vi "Telemetry Downlink Templates.vi"(11 "Command":T1 items=["Get xPG Status", "xPG Stimulation", "Select Program", "Increment Program Amplitude", "Decrement Program Amplitude", "Get PoP Constants", "Get PPC Constants", "Get Program Names", "Set Pulse Amplitude", "Increment Pulse Amplitude", "Decrement Pulse Amplitude", "Get Pulse Widths", "Set Pulse Widths", "Increment Pulse Width", "Decrement Pulse Width", "Get Program Frequency", "Set Program Frequency", "Increment Program Frequency", "Decrement Program Frequency", "Inject Event", "Charging Control", "Get xPG Identity", "Set xPG Identity", "Restore Program Defaults", "Get Program Definition", "Set Program Definition", "Get Program Constants", "Set Program Constants", "Get Configurable Device Parameters", "Set Configurable Device Parameters", "Get Pulse Constants", "Set Pulse Constants", "Get Lead Limits", "Set Lead Limits", "Get Channel Calibrations", "Set Channel Calibrations", "reserved", "reserved", "reserved", "reserved", "reserved", "reserved", "Get Stim Asic HV Calibrations", "Set Stim Asic HV Calibrations", "reserved", "reserved", "Get CP Data", "Set CP Data", "Clear Log", "Read Log", "Append Log", "Get Patient Program Runtime", "Set Patient Program Runtimec", "Impedance Measurement", "Enter Storage Mode", "Echo Short", "Echo Long", "Get General Calibration", "Set General Calibration", "Get Trim List", "Set Trim List", "Get Counter", "Set Counter", "Get Test Stimulation", "Set Test Stimulation", "Get Titration Stimulation", "Set Titration Stimulation", "Get Ramp Time", "Set Ramp Time", "Get VBAT", "Set Software Description Block", "Write Memory", "Read Memory", "Reset xPG", "Erase Flash Block", "Write Vectors", "Read Vectors", "Diagnostic Data", "Set Background Impedance", "Get Background Impedence ", "Undefined"]) -> (3 "Template String":string)   [LabVIEW 2010]
uses:
  Command List.ctl
panel:
  out "Token":u16 format="%05.0f"
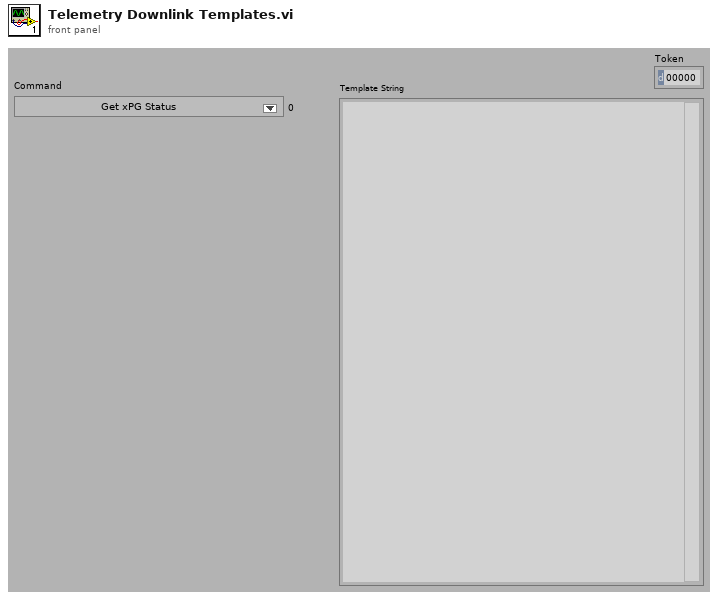
[diagram p1: front panel]
types:
  T1 = typedef "Command List.ctl" = u16
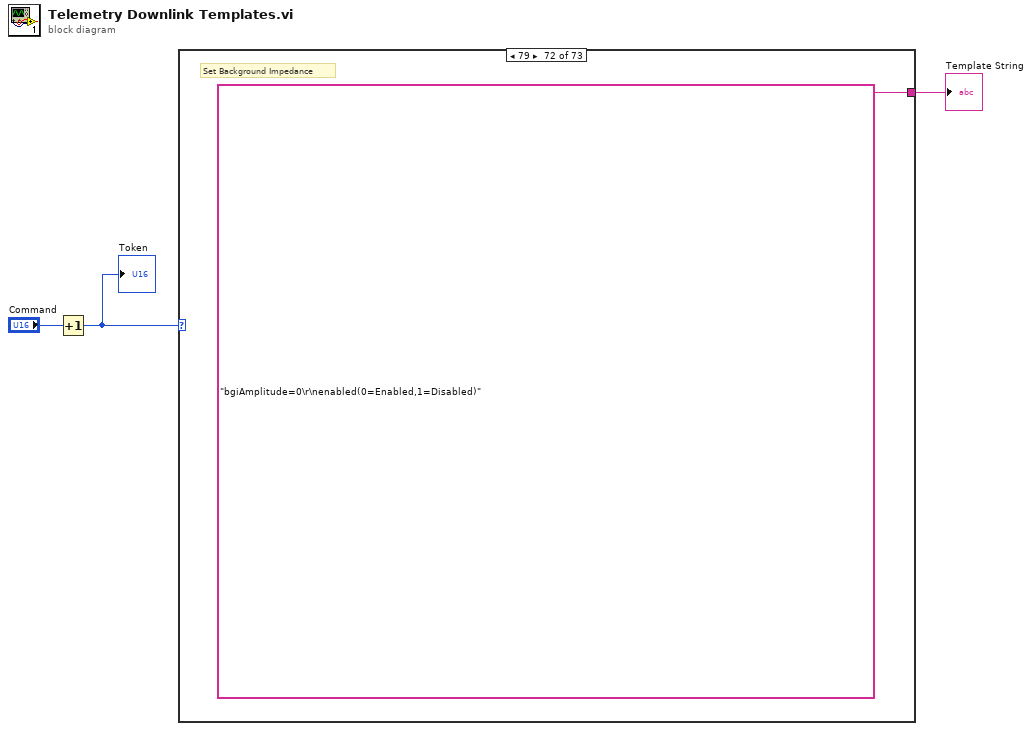
[diagram p0: block diagram]
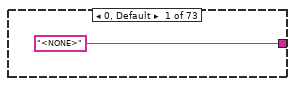
[diagram p2: hidden frame]
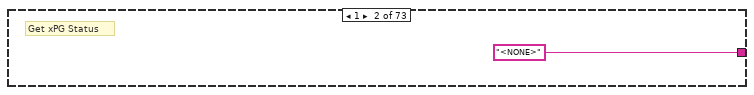
[diagram p3: hidden frame]
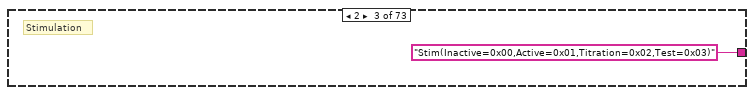
[diagram p4: hidden frame]
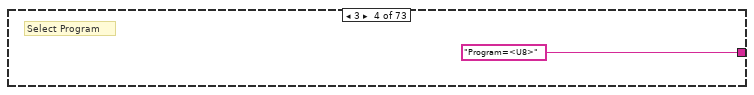
[diagram p5: hidden frame]
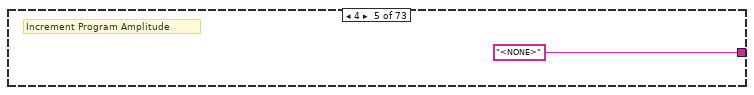
[diagram p6: hidden frame]
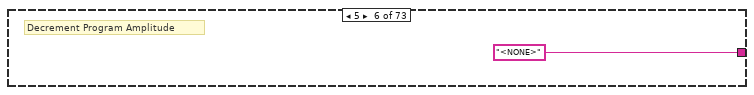
[diagram p7: hidden frame]
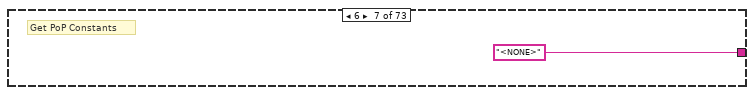
[diagram p8: hidden frame]
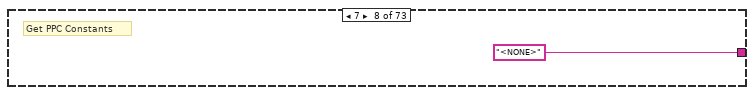
[diagram p9: hidden frame]
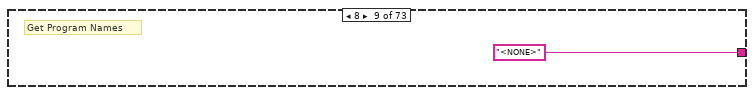
[diagram p10: hidden frame]
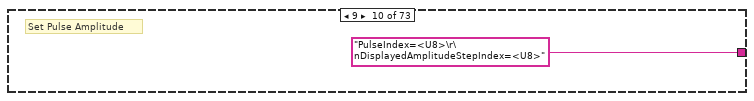
[diagram p11: hidden frame]
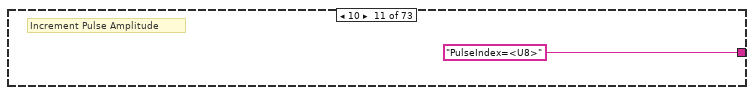
[diagram p12: hidden frame]
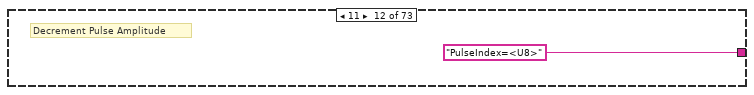
[diagram p13: hidden frame]
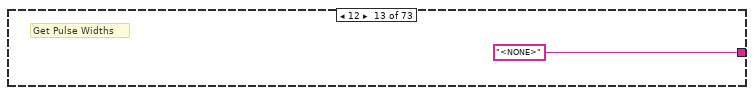
[diagram p14: hidden frame]
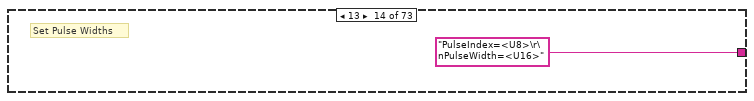
[diagram p15: hidden frame]
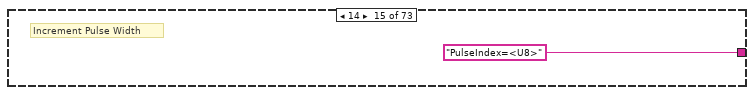
[diagram p16: hidden frame]
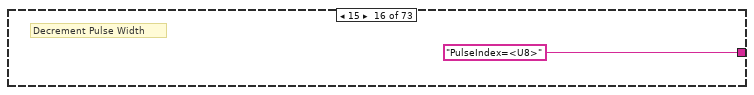
[diagram p17: hidden frame]
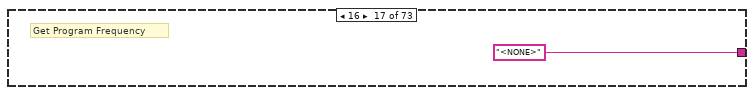
[diagram p18: hidden frame]
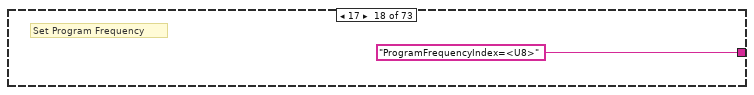
[diagram p19: hidden frame]
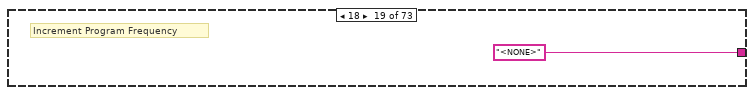
[diagram p20: hidden frame]
diagram:
  n1 = Increment(x="Command") -> (x+1=w2:T1)
  "Token" <- w2
  n2 = case shown="79" w2 {
    tunnel: ["<NONE>" "<NONE>" "Stim(Inactive=0x00,Active=0x01,Titration=0x02,Test=0x03)" "Program=<U8>" "<NONE>" "<NONE>" "<NONE>" "<NONE>" "<NONE>" "PulseIndex=<U8>\r\nDisplayedAmplitudeStepIndex=<U8>" "PulseIndex=<U8>" "PulseIndex=<U8>" "<NONE>" "PulseIndex=<U8>\r\nPulseWidth=<U16>" "PulseIndex=<U8>" "PulseIndex=<U8>" "<NONE>" "ProgramFrequencyIndex=<U8>" "<NONE>" "<NONE>" "eventID=<U16>\r\neventData=<U16>" "<NONE>" "<NONE>" "MICSID[1]=<U8>\r\nMICSID[2]=<U8>\r\nMICSID[3]=<U8>\r\nMICSID[4]=<U8>\r\nModelNumber=<String[10]>\r\nSerialNumber=<String[20]>" "RestoredProgramMap=<U16>" "Program=0" "ProgramNumber=0\nProgramDefined=0\nProgramDisabled=0\nProgramName=0\nAllowedFrequencies[0]=0x00\nAllowedFrequencies[1]=0x00\nAllowedFrequencies[2]=0x00\nAllowedFrequencies[3]=0x00\nAllowedFrequencies[4]=0x40\nAllowedFrequencies[5]=0x00\nAllowedFrequencies[6]=0x00\nAllowedFrequencies[7]=0x00\nProgramFrequencyIndex=0\nDefinedPulseMap=0\nPulseNamePA=0\nAmplitudeLowLimitPA=0\nAmplitudeStepPA=0\nAmplitudeStepIndexPA=0\nPulseWidthLowLimitPA=0\nPulseWidthHighLimitPA=0\nPulseWidthPA=0\nElectrodeAmpPercentagePA[CH01]=0\nElectrodeAmpPercentagePA[CH02]=0\nElectrodeAmpPercentagePA[CH03]=0\nElectrodeAmpPercentagePA[CH04]=0\nElectrodeAmpPercentagePA[CH05]=0\nElectrodeAmpPercentagePA[CH06]=0\nElectrodeAmpPercentagePA[CH07]=0\nElectrodeAmpPercentagePA[CH08]=0\nElectrodeAmpPercentagePA[CH09]=0\nElectrodeAmpPercentagePA[CH10]=0\nElectrodeAmpPercentagePA[CH11]=0\nElectrodeAmpPercentagePA[CH12]=0\nElectrodeAmpPercentagePA[CH13]=0\nElectrodeAmpPercentagePA[CH14]=0\nElectrodeAmpPercentagePA[CH15]=0\nElectrodeAmpPercentagePA[CH16]=0\nElectrodeAmpPercentagePA[CH17]=0\nElectrodeAmpPercentagePA[CH18]=0\nElectrodeAmpPercentagePA[CH19]=0\nElectrodeAmpPercentagePA[CH20]=0\nElectrodeAmpPercentagePA[CH21]=0\nElectrodeAmpPercentagePA[CH22]=0\nElectrodeAmpPercentagePA[CH23]=0\nElectrodeAmpPercentagePA[CH24]=0\nElectrodeAmpPercentagePA[CH25]=0\nElectrodeAmpPercentagePA[CH26]=0\nPulseNamePB=0\nAmplitudeLowLimitPB=0\nAmplitudeStepPB=0\nAmplitudeStepIndexPB=0\nPulseWidthLowLimitPB=0\nPulseWidthHighLimitPB=0\nPulseWidthPB=0\nElectrodeAmpPercentagePB[CH01]=0\nElectrodeAmpPercentagePB[CH02]=0\nElectrodeAmpPercentagePB[CH03]=0\nElectrodeAmpPercentagePB[CH04]=0\nElectrodeAmpPercentagePB[CH05]=0\nElectrodeAmpPercentagePB[CH06]=0\nElectrodeAmpPercentagePB[CH07]=0\nElectrodeAmpPercentagePB[CH08]=0\nElectrodeAmpPercentagePB[CH09]=0\nElectrodeAmpPercentagePB[CH10]=0\nElectrodeAmpPercentagePB[CH11]=0\nElectrodeAmpPercentagePB[CH12]=0\nElectrodeAmpPercentagePB[CH13]=0\nElectrodeAmpPercentagePB[CH14]=0\nElectrodeAmpPercentagePB[CH15]=0\nElectrodeAmpPercentagePB[CH16]=0\nElectrodeAmpPercentagePB[CH17]=0\nElectrodeAmpPercentagePB[CH18]=0\nElectrodeAmpPercentagePB[CH19]=0\nElectrodeAmpPercentagePB[CH20]=0\nElectrodeAmpPercentagePB[CH21]=0\nElectrodeAmpPercentagePB[CH22]=0\nElectrodeAmpPercentagePB[CH23]=0\nElectrodeAmpPercentagePB[CH24]=0\nElectrodeAmpPercentagePB[CH25]=0\nElectrodeAmpPercentagePB[CH26]=0\nPulseNamePC=0\nAmplitudeLowLimitPC=0\nAmplitudeStepPC=0\nAmplitudeStepIndexPC=0\nPulseWidthLowLimitPC=0\nPulseWidthHighLimitPC=0\nPulseWidthPC=0\nElectrodeAmpPercentagePC[CH01]=0\nElectrodeAmpPercentagePC[CH02]=0\nElectrodeAmpPercentagePC[CH03]=0\nElectrodeAmpPercentagePC[CH04]=0\nElectrodeAmpPercentagePC[CH05]=0\nElectrodeAmpPercentagePC[CH06]=0\nElectrodeAmpPercentagePC[CH07]=0\nElectrodeAmpPercentagePC[CH08]=0\nElectrodeAmpPercentagePC[CH09]=0\nElectrodeAmpPercentagePC[CH10]=0\nElectrodeAmpPercentagePC[CH11]=0\nElectrodeAmpPercentagePC[CH12]=0\nElectrodeAmpPercentagePC[CH13]=0\nElectrodeAmpPercentagePC[CH14]=0\nElectrodeAmpPercentagePC[CH15]=0\nElectrodeAmpPercentagePC[CH16]=0\nElectrodeAmpPercentagePC[CH17]=0\nElectrodeAmpPercentagePC[CH18]=0\nElectrodeAmpPercentagePC[CH19]=0\nElectrodeAmpPercentagePC[CH20]=0\nElectrodeAmpPercentagePC[CH21]=0\nElectrodeAmpPercentagePC[CH22]=0\nElectrodeAmpPercentagePC[CH23]=0\nElectrodeAmpPercentagePC[CH24]=0\nElectrodeAmpPercentagePC[CH25]=0\nElectrodeAmpPercentagePC[CH26]=0\nPulseNamePD=0\nAmplitudeLowLimitPD=0\nAmplitudeStepPD=0\nAmplitudeStepIndexPD=0\nPulseWidthLowLimitPD=0\nPulseWidthHighLimitPD=0\nPulseWidthPD=0\nElectrodeAmpPercentagePD[CH01]=0\nElectrodeAmpPercentagePD[CH02]=0\nElectrodeAmpPercentagePD[CH03]=0\nElectrodeAmpPercentagePD[CH04]=0\nElectrodeAmpPercentagePD[CH05]=0\nElectrodeAmpPercentagePD[CH06]=0\nElectrodeAmpPercentagePD[CH07]=0\nElectrodeAmpPercentagePD[CH08]=0\nElectrodeAmpPercentagePD[CH09]=0\nElectrodeAmpPercentagePD[CH10]=0\nElectrodeAmpPercentagePD[CH11]=0\nElectrodeAmpPercentagePD[CH12]=0\nElectrodeAmpPercentagePD[CH13]=0\nElectrodeAmpPercentagePD[CH14]=0\nElectrodeAmpPercentagePD[CH15]=0\nElectrodeAmpPercentagePD[CH16]=0\nElectrodeAmpPercentagePD[CH17]=0\nElectrodeAmpPercentagePD[CH18]=0\nElectrodeAmpPercentagePD[CH19]=0\nElectrodeAmpPercentagePD[CH20]=0\nElectrodeAmpPercentagePD[CH21]=0\nElectrodeAmpPercentagePD[CH22]=0\nElectrodeAmpPercentagePD[CH23]=0\nElectrodeAmpPercentagePD[CH24]=0\nElectrodeAmpPercentagePD[CH25]=0\nElectrodeAmpPercentagePD[CH26]=0" "<NONE>" "RampTime=<U16>\r\nProgramFrequencies[00]=<U16>\r\nProgramFrequencies[01]=<U16>\r\nProgramFrequencies[02]=<U16>\r\nProgramFrequencies[03]=<U16>\r\nProgramFrequencies[04]=<U16>\r\nProgramFrequencies[05]=<U16>\r\nProgramFrequencies[06]=<U16>\r\nProgramFrequencies[07]=<U16>\r\nProgramFrequencies[08]=<U16>\r\nProgramFrequencies[09]=<U16>\r\nProgramFrequencies[10]=<U16>\r\nProgramFrequencies[11]=<U16>\r\nProgramFrequencies[12]=<U16>\r\nProgramFrequencies[13]=<U16>\r\nProgramFrequencies[14]=<U16>\r\nProgramFrequencies[15]=<U16>\r\nProgramFrequencies[16]=<U16>\r\nProgramFrequencies[17]=<U16>\r\nProgramFrequencies[18]=<U16>\r\nProgramFrequencies[19]=<U16>\r\nProgramFrequencies[20]=<U16>\r\nProgramFrequencies[21]=<U16>\r\nProgramFrequencies[22]=<U16>\r\nProgramFrequencies[23]=<U16>\r\nProgramFrequencies[24]=<U16>\r\nProgramFrequencies[25]=<U16>\r\nProgramFrequencies[26]=<U16>\r\nProgramFrequencies[27]=<U16>\r\nProgramFrequencies[28]=<U16>\r\nProgramFrequencies[29]=<U16>\r\nProgramFrequencies[30]=<U16>\r\nProgramFrequencies[31]=<U16>\r\nProgramFrequencies[32]=<U16>\r\nProgramFrequencies[33]=<U16>\r\nProgramFrequencies[34]=<U16>\r\nProgramFrequencies[35]=<U16>\r\nProgramFrequencies[36]=<U16>\r\nProgramFrequencies[37]=<U16>\r\nProgramFrequencies[38]=<U16>\r\nProgramFrequencies[39]=<U16>\r\nProgramFrequencies[40]=<U16>\r\nProgramFrequencies[41]=<U16>\r\nProgramFrequencies[42]=<U16>\r\nProgramFrequencies[43]=<U16>\r\nProgramFrequencies[44]=<U16>\r\nProgramFrequencies[45]=<U16>\r\nProgramFrequencies[46]=<U16>\r\nProgramFrequencies[47]=<U16>\r\nProgramFrequencies[48]=<U16>\r\nProgramFrequencies[49]=<U16>\r\nProgramFrequencies[50]=<U16>\r\nProgramFrequencies[51]=<U16>\r\nProgramFrequencies[52]=<U16>\r\nProgramFrequencies[53]=<U16>\r\nProgramFrequencies[54]=<U16>\r\nProgramFrequencies[55]=<U16>\r\nProgramFrequencies[56]=<U16>\r\nProgramFrequencies[57]=<U16>\r\nProgramFrequencies[58]=<U16>\r\nProgramFrequencies[59]=<U16>\r\nProgramFrequencies[60]=<U16>\r\nProgramFrequencies[61]=<U16>\r\nProgramFrequencies[62]=<U16>\r\nProgramFrequencies[63]=<U16>" "<NONE>" "PPC_Enabled=<U8>\r\nPPC_EXID[0]=<U8>\r\nPPC_EXID[1]=<U8>\r\nPPC_EXID[2]=<U8>\r\nPOP1_Enabled=<U8>\r\nPOP1_EXID[0]=<U8>\r\nPOP1_EXID[1]=<U8>\r\nPOP1_EXID[2]=<U8>\r\nPOP2_Enabled=<U8>\r\nPOP2_EXID[0]=<U8>\r\nPOP2_EXID[1]=<U8>\r\nPOP2_EXID[2]=<U8>\r\nPPC_Text=<String[30]>\r\nPulseWidthStep=<U16>\r\nAmplitudeSteps=<U8>\r\nPPC_Options=<U8>\r\nIPG_Magnet_Options=<U8>\r\nImplantDateTime=<MM/DD/YYYY 00=00=00>\r\nReplacementIntervalMonths=<U8>" "<NONE>" "PassiveInterphaseDelay=0\nPassiveRecoveryWidth=0\nPassiveRecoveryHoldoff=0\nPassiveCBCWidth=0\nPassiveCBCHoldoff=0\nActiveInterphaseDelay=0\nActiveRecoveryHoldoff=0\nActiveCBCWidth=0\nActiveCBCHoldoff=0\nKrecsEnabledBitMap=0\nIncrementLockoutMsecs=0\nStimPhasePSDisableActive=0\nUncontrolledSourceSinkEnabled=0" "<NONE>" "currentLimit[CH01]=0\ncurrentLimit[CH02]=0\ncurrentLimit[CH03]=0\ncurrentLimit[CH04]=0\ncurrentLimit[CH05]=0\ncurrentLimit[CH06]=0\ncurrentLimit[CH07]=0\ncurrentLimit[CH08]=0\ncurrentLimit[CH09]=0\ncurrentLimit[CH10]=0\ncurrentLimit[CH11]=0\ncurrentLimit[CH12]=0\ncurrentLimit[CH13]=0\ncurrentLimit[CH14]=0\ncurrentLimit[CH15]=0\ncurrentLimit[CH16]=0\ncurrentLimit[CH17]=0\ncurrentLimit[CH18]=0\ncurrentLimit[CH19]=0\ncurrentLimit[CH20]=0\ncurrentLimit[CH21]=0\ncurrentLimit[CH22]=0\ncurrentLimit[CH23]=0\ncurrentLimit[CH24]=0\ncurrentLimit[CH25]=0\ncurrentLimit[CH26]=0\nchargeLimit[CH01]=0\nchargeLimit[CH02]=0\nchargeLimit[CH03]=0\nchargeLimit[CH04]=0\nchargeLimit[CH05]=0\nchargeLimit[CH06]=0\nchargeLimit[CH07]=0\nchargeLimit[CH08]=0\nchargeLimit[CH09]=0\nchargeLimit[CH10]=0\nchargeLimit[CH11]=0\nchargeLimit[CH12]=0\nchargeLimit[CH13]=0\nchargeLimit[CH14]=0\nchargeLimit[CH15]=0\nchargeLimit[CH16]=0\nchargeLimit[CH17]=0\nchargeLimit[CH18]=0\nchargeLimit[CH19]=0\nchargeLimit[CH20]=0\nchargeLimit[CH21]=0\nchargeLimit[CH22]=0\nchargeLimit[CH23]=0\nchargeLimit[CH24]=0\nchargeLimit[CH25]=0\nchargeLimit[CH26]=0" "<NONE>" "channelCalSourcing[CH01]=<U16>\r\nchannelCalSourcing[CH02]=<U16>\r\nchannelCalSourcing[CH03]=<U16>\r\nchannelCalSourcing[CH04]=<U16>\r\nchannelCalSourcing[CH05]=<U16>\r\nchannelCalSourcing[CH06]=<U16>\r\nchannelCalSourcing[CH07]=<U16>\r\nchannelCalSourcing[CH08]=<U16>\r\nchannelCalSourcing[CH09]=<U16>\r\nchannelCalSourcing[CH10]=<U16>\r\nchannelCalSourcing[CH11]=<U16>\r\nchannelCalSourcing[CH12]=<U16>\r\nchannelCalSourcing[CH13]=<U16>\r\nchannelCalSourcing[CH14]=<U16>\r\nchannelCalSourcing[CH15]=<U16>\r\nchannelCalSourcing[CH16]=<U16>\r\nchannelCalSourcing[CH17]=<U16>\r\nchannelCalSourcing[CH18]=<U16>\r\nchannelCalSourcing[CH19]=<U16>\r\nchannelCalSourcing[CH20]=<U16>\r\nchannelCalSourcing[CH21]=<U16>\r\nchannelCalSourcing[CH22]=<U16>\r\nchannelCalSourcing[CH23]=<U16>\r\nchannelCalSourcing[CH24]=<U16>\r\nchannelCalSourcing[CH25]=<U16>\r\nchannelCalSourcing[CH26]=<U16>\r\nchannelCalSinking[CH01]=<U16>\r\nchannelCalSinking[CH02]=<U16>\r\nchannelCalSinking[CH03]=<U16>\r\nchannelCalSinking[CH04]=<U16>\r\nchannelCalSinking[CH05]=<U16>\r\nchannelCalSinking[CH06]=<U16>\r\nchannelCalSinking[CH07]=<U16>\r\nchannelCalSinking[CH08]=<U16>\r\nchannelCalSinking[CH09]=<U16>\r\nchannelCalSinking[CH10]=<U16>\r\nchannelCalSinking[CH11]=<U16>\r\nchannelCalSinking[CH12]=<U16>\r\nchannelCalSinking[CH13]=<U16>\r\nchannelCalSinking[CH14]=<U16>\r\nchannelCalSinking[CH15]=<U16>\r\nchannelCalSinking[CH16]=<U16>\r\nchannelCalSinking[CH17]=<U16>\r\nchannelCalSinking[CH18]=<U16>\r\nchannelCalSinking[CH19]=<U16>\r\nchannelCalSinking[CH20]=<U16>\r\nchannelCalSinking[CH21]=<U16>\r\nchannelCalSinking[CH22]=<U16>\r\nchannelCalSinking[CH23]=<U16>\r\nchannelCalSinking[CH24]=<U16>\r\nchannelCalSinking[CH25]=<U16>\r\nchannelCalSinking[CH26]=<U16>" "<NONE>" "stimAsicHVmVOutput[00]=<U16>\r\nstimAsicHVmVOutput[01]=<U16>\r\nstimAsicHVmVOutput[02]=<U16>\r\nstimAsicHVmVOutput[03]=<U16>\r\nstimAsicHVmVOutput[04]=<U16>\r\nstimAsicHVmVOutput[05]=<U16>\r\nstimAsicHVmVOutput[06]=<U16>\r\nstimAsicHVmVOutput[07]=<U16>\r\nstimAsicHVmVOutput[08]=<U16>\r\nstimAsicHVmVOutput[09]=<U16>\r\nstimAsicHVmVOutput[10]=<U16>\r\nstimAsicHVmVOutput[11]=<U16>\r\nstimAsicHVmVOutput[12]=<U16>\r\nstimAsicHVmVOutput[13]=<U16>\r\nstimAsicHVmVOutput[14]=<U16>\r\nstimAsicHVmVOutput[15]=<U16>\r\nstimAsicHVmVOutput[16]=<U16>\r\nstimAsicHVmVOutput[17]=<U16>\r\nstimAsicHVmVOutput[18]=<U16>\r\nstimAsicHVmVOutput[19]=<U16>\r\nstimAsicHVmVOutput[20]=<U16>\r\nstimAsicHVmVOutput[21]=<U16>\r\nstimAsicHVmVOutput[22]=<U16>\r\nstimAsicHVmVOutput[23]=<U16>\r\nstimAsicHVmVOutput[24]=<U16>\r\nstimAsicHVmVOutput[25]=<U16>\r\nstimAsicHVmVOutput[26]=<U16>\r\nstimAsicHVmVOutput[27]=<U16>\r\nstimAsicHVmVOutput[28]=<U16>\r\nstimAsicHVmVOutput[29]=<U16>\r\nstimAsicHVmVOutput[30]=<U16>\r\nstimAsicHVmVOutput[31]=<U16>\r\nstimAsicHVmVOutput[32]=<U16>\r\nstimAsicHVmVOutput[33]=<U16>\r\nstimAsicHVmVOutput[34]=<U16>\r\nstimAsicHVmVOutput[35]=<U16>\r\nstimAsicHVmVOutput[36]=<U16>\r\nstimAsicHVmVOutput[37]=<U16>\r\nstimAsicHVmVOutput[38]=<U16>\r\nstimAsicHVmVOutput[39]=<U16>\r\nstimAsicHVmVOutput[40]=<U16>\r\nstimAsicHVmVOutput[41]=<U16>\r\nstimAsicHVmVOutput[42]=<U16>\r\nstimAsicHVmVOutput[43]=<U16>\r\nstimAsicHVmVOutput[44]=<U16>\r\nstimAsicHVmVOutput[45]=<U16>\r\nstimAsicHVmVOutput[46]=<U16>\r\nstimAsicHVmVOutput[47]=<U16>\r\nstimAsicHVmVOutput[48]=<U16>\r\nstimAsicHVmVOutput[49]=<U16>\r\nstimAsicHVmVOutput[50]=<U16>\r\nstimAsicHVmVOutput[51]=<U16>\r\nstimAsicHVmVOutput[52]=<U16>\r\nstimAsicHVmVOutput[53]=<U16>\r\nstimAsicHVmVOutput[54]=<U16>\r\nstimAsicHVmVOutput[55]=<U16>\r\nstimAsicHVmVOutput[56]=<U16>\r\nstimAsicHVmVOutput[57]=<U16>\r\nstimAsicHVmVOutput[58]=<U16>\r\nstimAsicHVmVOutput[59]=<U16>\r\nstimAsicHVmVOutput[60]=<U16>\r\nstimAsicHVmVOutput[61]=<U16>\r\nstimAsicHVmVOutput[62]=<U16>\r\nstimAsicHVmVOutput[63]=<U16>" "CPDataBlockSelect=<U8>" "CPDataBlockSelect=<U8>\r\n<U8 Array[256]>" "LogNum=0" "LogNum=0\r\nSerial=0" "LogNum=\nEvent=\r\nEventData[0]=\r\nEventData[1]=\r\nEventData[2]=\r\nEventData[3]=" "patientProgramNumber=<U8>" "patientProgramNumber=<U8>\r\npatientProgramRunTime=<U32>" "channel_A=<U8>\r\nchannel_B=<U8>\r\nmeasurementPulseAmplitude=<U16>\r\nmeasurementPulseWidth=<U16>\r\nmeasurementPulseInterphaseDelay=<U16>\r\nmeasurementPulsePassiveRecoveryWidth=<U16>\r\nmeasurementPulseRecoveryHoldoff=<U16>\r\nmeasurementPulseFrequency=<U16>\r\nnumberofpulses=<U8>" "<NONE>" "Data = 1st 8 bytes of CP_DATA" "Data =9 or more bytes of CP_DATA" "<NONE>" "Reserved[00]=<U16>\r\nReserved[01]=<U16>\r\nReserved[02]=<U16>\r\nReserved[03]=<U16>\r\nReserved[04]=<U16>\r\nReserved[05]=<U16>\r\nReserved[06]=<U16>\r\nReserved[07]=<U16>\r\nReserved[08]=<U16>\r\nReserved[09]=<U16>\r\nReserved[10]=<U16>\r\nReserved[11]=<U16>\r\nReserved[12]=<U16>\r\nReserved[13]=<U16>\r\nReserved[14]=<U16>\r\ntempMinThreshold=<U16>\r\ntempWarningThresholdl=<U16>\r\ntempCriticalThresholdl=<U16>\r\ntempAbortThresholdl=<U16>\r\nthermOffsetMinimum=<U16>\r\nthermOffsetMaximum=<U16>\r\nthermBiasMinimum=<U16>\r\nthermBiasMaximum=<U16>\r\nthermInputMinimum=<U16>\r\nthermInputMaximum=<U16>\r\nbatteryIncreasePreCharge=<U16>\r\nbatteryIncreaseConstandCurrent=<U16>\r\nReserved[00]=<U16>\r\nReserved[01]=<U16>\r\nReserved[02]=<U16>\r\nReserved[03]=<U16>\r\nReserved[04]=<U16>\r\nReserved[05]=<U16>\r\nReserved[06]=<U16>\r\nReserved[07]=<U16>\r\nReserved[08]=<U16>\r\nReserved[09]=<U16>\r\nReserved[10]=<U16>\r\nReserved[11]=<U16>\r\nReserved[12]=<U16>\r\nReserved[13]=<U16>\r\nReserved[14]=<U16>\r\nbatteryStateCalStimOff[00]=<U16>\r\nbatteryStateCalStimOff[01]=<U16>\r\nbatteryStateCalStimOff[02]=<U16>\r\nbatteryStateCalStimOff[03]=<U16>\r\nbatteryStateCalStimOff[04]=<U16>\r\nbatteryStateCalStimOff[05]=<U16>\r\nbatteryStateCalStimOn[00]=<U16>\r\nbatteryStateCalStimOn[01]=<U16>\r\nbatteryStateCalStimOn[02]=<U16>\r\nbatteryStateCalStimOn[03]=<U16>\r\nbatteryStateCalStimOn[04]=<U16>\r\nbatteryStateCalStimOn[05]=<U16>\r\nvrectMeasurementCal=<U16>" "ListNum(0=PWR,1=MICS,2=STIM)=<U8>" "ListNum(0=PWR,1=MICS,2=STIM)=<U8>\r\nListLen=<U8>\r\nAddress=<U16>\r\nData=<U8>\r\n\r\n*Duplicate \"Address\" and \"Data\" pairs for #ListLen data entries, then remove this comment line.*" "eventCounterID=<U8>" "eventCounterID=<U8>\r\neventCount=<U16>" "<NONE>" "FrequencyIndex=<U8>\r\nComplianceVoltage=<U8>\r\nNumPulses=<U8>\r\nAmplitudePA=<U16>\r\nchannelPercentagePA[CH01]=<I8>\r\nchannelPercentagePA[CH02]=<I8>\r\nchannelPercentagePA[CH03]=<I8>\r\nchannelPercentagePA[CH04]=<I8>\r\nchannelPercentagePA[CH05]=<I8>\r\nchannelPercentagePA[CH06]=<I8>\r\nchannelPercentagePA[CH07]=<I8>\r\nchannelPercentagePA[CH08]=<I8>\r\nchannelPercentagePA[CH09]=<I8>\r\nchannelPercentagePA[CH10]=<I8>\r\nchannelPercentagePA[CH11]=<I8>\r\nchannelPercentagePA[CH12]=<I8>\r\nchannelPercentagePA[CH13]=<I8>\r\nchannelPercentagePA[CH14]=<I8>\r\nchannelPercentagePA[CH15]=<I8>\r\nchannelPercentagePA[CH16]=<I8>\r\nchannelPercentagePA[CH17]=<I8>\r\nchannelPercentagePA[CH18]=<I8>\r\nchannelPercentagePA[CH19]=<I8>\r\nchannelPercentagePA[CH20]=<I8>\r\nchannelPercentagePA[CH21]=<I8>\r\nchannelPercentagePA[CH22]=<I8>\r\nchannelPercentagePA[CH23]=<I8>\r\nchannelPercentagePA[CH24]=<I8>\r\nchannelPercentagePA[CH25]=<I8>\r\nchannelPercentagePA[CH26]=<I8>\r\nStimWidthPA=<U16>\r\nInterphaseDelayPA=<U8>\r\nRecoveryRatioSelectPA=<U8>\r\nPassiveRecoveryWidthPA=<U16>\r\nCBCWidthPA=<U16>\r\nFlags(01=Stim,02=Rec,04=Cbc)PA=<U8>\r\nAmplitudePB=<U16>\r\nchannelPercentagePB[CH01]=<I8>\r\nchannelPercentagePB[CH02]=<I8>\r\nchannelPercentagePB[CH03]=<I8>\r\nchannelPercentagePB[CH04]=<I8>\r\nchannelPercentagePB[CH05]=<I8>\r\nchannelPercentagePB[CH06]=<I8>\r\nchannelPercentagePB[CH07]=<I8>\r\nchannelPercentagePB[CH08]=<I8>\r\nchannelPercentagePB[CH09]=<I8>\r\nchannelPercentagePB[CH10]=<I8>\r\nchannelPercentagePB[CH11]=<I8>\r\nchannelPercentagePB[CH12]=<I8>\r\nchannelPercentagePB[CH13]=<I8>\r\nchannelPercentagePB[CH14]=<I8>\r\nchannelPercentagePB[CH15]=<I8>\r\nchannelPercentagePB[CH16]=<I8>\r\nchannelPercentagePB[CH17]=<I8>\r\nchannelPercentagePB[CH18]=<I8>\r\nchannelPercentagePB[CH19]=<I8>\r\nchannelPercentagePB[CH20]=<I8>\r\nchannelPercentagePB[CH21]=<I8>\r\nchannelPercentagePB[CH22]=<I8>\r\nchannelPercentagePB[CH23]=<I8>\r\nchannelPercentagePB[CH24]=<I8>\r\nchannelPercentagePB[CH25]=<I8>\r\nchannelPercentagePB[CH26]=<I8>\r\nStimWidthPB=<U16>\r\nInterphaseDelayPB=<U8>\r\nRecoveryRatioSelectPB=<U8>\r\nPassiveRecoveryWidthPB=<U16>\r\nCBCWidthPB=<U16>\r\nFlags(01=Stim,02=Rec,04=Cbc)PB=<U8>\r\nAmplitudePC=<U16>\r\nchannelPercentagePC[CH01]=<I8>\r\nchannelPercentagePC[CH02]=<I8>\r\nchannelPercentagePC[CH03]=<I8>\r\nchannelPercentagePC[CH04]=<I8>\r\nchannelPercentagePC[CH05]=<I8>\r\nchannelPercentagePC[CH06]=<I8>\r\nchannelPercentagePC[CH07]=<I8>\r\nchannelPercentagePC[CH08]=<I8>\r\nchannelPercentagePC[CH09]=<I8>\r\nchannelPercentagePC[CH10]=<I8>\r\nchannelPercentagePC[CH11]=<I8>\r\nchannelPercentagePC[CH12]=<I8>\r\nchannelPercentagePC[CH13]=<I8>\r\nchannelPercentagePC[CH14]=<I8>\r\nchannelPercentagePC[CH15]=<I8>\r\nchannelPercentagePC[CH16]=<I8>\r\nchannelPercentagePC[CH17]=<I8>\r\nchannelPercentagePC[CH18]=<I8>\r\nchannelPercentagePC[CH19]=<I8>\r\nchannelPercentagePC[CH20]=<I8>\r\nchannelPercentagePC[CH21]=<I8>\r\nchannelPercentagePC[CH22]=<I8>\r\nchannelPercentagePC[CH23]=<I8>\r\nchannelPercentagePC[CH24]=<I8>\r\nchannelPercentagePC[CH25]=<I8>\r\nchannelPercentagePC[CH26]=<I8>\r\nStimWidthPC=<U16>\r\nInterphaseDelayPC=<U8>\r\nRecoveryRatioSelectPC=<U8>\r\nPassiveRecoveryWidthPC=<U16>\r\nCBCWidthPC=<U16>\r\nFlags(01=Stim,02=Rec,04=Cbc)PC=<U8>\r\nAmplitudePD=<U16>\r\nchannelPercentagePD[CH01]=<I8>\r\nchannelPercentagePD[CH02]=<I8>\r\nchannelPercentagePD[CH03]=<I8>\r\nchannelPercentagePD[CH04]=<I8>\r\nchannelPercentagePD[CH05]=<I8>\r\nchannelPercentagePD[CH06]=<I8>\r\nchannelPercentagePD[CH07]=<I8>\r\nchannelPercentagePD[CH08]=<I8>\r\nchannelPercentagePD[CH09]=<I8>\r\nchannelPercentagePD[CH10]=<I8>\r\nchannelPercentagePD[CH11]=<I8>\r\nchannelPercentagePD[CH12]=<I8>\r\nchannelPercentagePD[CH13]=<I8>\r\nchannelPercentagePD[CH14]=<I8>\r\nchannelPercentagePD[CH15]=<I8>\r\nchannelPercentagePD[CH16]=<I8>\r\nchannelPercentagePD[CH17]=<I8>\r\nchannelPercentagePD[CH18]=<I8>\r\nchannelPercentagePD[CH19]=<I8>\r\nchannelPercentagePD[CH20]=<I8>\r\nchannelPercentagePD[CH21]=<I8>\r\nchannelPercentagePD[CH22]=<I8>\r\nchannelPercentagePD[CH23]=<I8>\r\nchannelPercentagePD[CH24]=<I8>\r\nchannelPercentagePD[CH25]=<I8>\r\nchannelPercentagePD[CH26]=<I8>\r\nStimWidthPD=<U16>\r\nInterphaseDelayPD=<U8>\r\nRecoveryRatioSelectPD=<U8>\r\nPassiveRecoveryWidthPD=<U16>\r\nCBCWidthPD=<U16>\r\nFlags(01=Stim,02=Rec,04=Cbc)PD=<U8>" "<NONE>" "frequencyIndex=<U8>\r\nnumPulses=<U8>\r\nAmplitudePA=<U16>\r\npulseWidthPA=<U16>\r\nchannelPercentagePA[CH01]=<I8>\r\nchannelPercentagePA[CH02]=<I8>\r\nchannelPercentagePA[CH03]=<I8>\r\nchannelPercentagePA[CH04]=<I8>\r\nchannelPercentagePA[CH05]=<I8>\r\nchannelPercentagePA[CH06]=<I8>\r\nchannelPercentagePA[CH07]=<I8>\r\nchannelPercentagePA[CH08]=<I8>\r\nchannelPercentagePA[CH09]=<I8>\r\nchannelPercentagePA[CH10]=<I8>\r\nchannelPercentagePA[CH11]=<I8>\r\nchannelPercentagePA[CH12]=<I8>\r\nchannelPercentagePA[CH13]=<I8>\r\nchannelPercentagePA[CH14]=<I8>\r\nchannelPercentagePA[CH15]=<I8>\r\nchannelPercentagePA[CH16]=<I8>\r\nchannelPercentagePA[CH17]=<I8>\r\nchannelPercentagePA[CH18]=<I8>\r\nchannelPercentagePA[CH19]=<I8>\r\nchannelPercentagePA[CH20]=<I8>\r\nchannelPercentagePA[CH21]=<I8>\r\nchannelPercentagePA[CH22]=<I8>\r\nchannelPercentagePA[CH23]=<I8>\r\nchannelPercentagePA[CH24]=<I8>\r\nchannelPercentagePA[CH25]=<I8>\r\nchannelPercentagePA[CH26]=<I8>\r\nAmplitudePB=<U16>\r\npulseWidthPB=<U16>\r\nchannelPercentagePB[CH01]=<I8>\r\nchannelPercentagePB[CH02]=<I8>\r\nchannelPercentagePB[CH03]=<I8>\r\nchannelPercentagePB[CH04]=<I8>\r\nchannelPercentagePB[CH05]=<I8>\r\nchannelPercentagePB[CH06]=<I8>\r\nchannelPercentagePB[CH07]=<I8>\r\nchannelPercentagePB[CH08]=<I8>\r\nchannelPercentagePB[CH09]=<I8>\r\nchannelPercentagePB[CH10]=<I8>\r\nchannelPercentagePB[CH11]=<I8>\r\nchannelPercentagePB[CH12]=<I8>\r\nchannelPercentagePB[CH13]=<I8>\r\nchannelPercentagePB[CH14]=<I8>\r\nchannelPercentagePB[CH15]=<I8>\r\nchannelPercentagePB[CH16]=<I8>\r\nchannelPercentagePB[CH17]=<I8>\r\nchannelPercentagePB[CH18]=<I8>\r\nchannelPercentagePB[CH19]=<I8>\r\nchannelPercentagePB[CH20]=<I8>\r\nchannelPercentagePB[CH21]=<I8>\r\nchannelPercentagePB[CH22]=<I8>\r\nchannelPercentagePB[CH23]=<I8>\r\nchannelPercentagePB[CH24]=<I8>\r\nchannelPercentagePB[CH25]=<I8>\r\nchannelPercentagePB[CH26]=<I8>\r\nAmplitudePC=<U16>\r\npulseWidthPC=<U16>\r\nchannelPercentagePC[CH01]=<I8>\r\nchannelPercentagePC[CH02]=<I8>\r\nchannelPercentagePC[CH03]=<I8>\r\nchannelPercentagePC[CH04]=<I8>\r\nchannelPercentagePC[CH05]=<I8>\r\nchannelPercentagePC[CH06]=<I8>\r\nchannelPercentagePC[CH07]=<I8>\r\nchannelPercentagePC[CH08]=<I8>\r\nchannelPercentagePC[CH09]=<I8>\r\nchannelPercentagePC[CH10]=<I8>\r\nchannelPercentagePC[CH11]=<I8>\r\nchannelPercentagePC[CH12]=<I8>\r\nchannelPercentagePC[CH13]=<I8>\r\nchannelPercentagePC[CH14]=<I8>\r\nchannelPercentagePC[CH15]=<I8>\r\nchannelPercentagePC[CH16]=<I8>\r\nchannelPercentagePC[CH17]=<I8>\r\nchannelPercentagePC[CH18]=<I8>\r\nchannelPercentagePC[CH19]=<I8>\r\nchannelPercentagePC[CH20]=<I8>\r\nchannelPercentagePC[CH21]=<I8>\r\nchannelPercentagePC[CH22]=<I8>\r\nchannelPercentagePC[CH23]=<I8>\r\nchannelPercentagePC[CH24]=<I8>\r\nchannelPercentagePC[CH25]=<I8>\r\nchannelPercentagePC[CH26]=<I8>\r\nAmplitudePD=<U16>\r\npulseWidthPD=<U16>\r\nchannelPercentagePD[CH01]=<I8>\r\nchannelPercentagePD[CH02]=<I8>\r\nchannelPercentagePD[CH03]=<I8>\r\nchannelPercentagePD[CH04]=<I8>\r\nchannelPercentagePD[CH05]=<I8>\r\nchannelPercentagePD[CH06]=<I8>\r\nchannelPercentagePD[CH07]=<I8>\r\nchannelPercentagePD[CH08]=<I8>\r\nchannelPercentagePD[CH09]=<I8>\r\nchannelPercentagePD[CH10]=<I8>\r\nchannelPercentagePD[CH11]=<I8>\r\nchannelPercentagePD[CH12]=<I8>\r\nchannelPercentagePD[CH13]=<I8>\r\nchannelPercentagePD[CH14]=<I8>\r\nchannelPercentagePD[CH15]=<I8>\r\nchannelPercentagePD[CH16]=<I8>\r\nchannelPercentagePD[CH17]=<I8>\r\nchannelPercentagePD[CH18]=<I8>\r\nchannelPercentagePD[CH19]=<I8>\r\nchannelPercentagePD[CH20]=<I8>\r\nchannelPercentagePD[CH21]=<I8>\r\nchannelPercentagePD[CH22]=<I8>\r\nchannelPercentagePD[CH23]=<I8>\r\nchannelPercentagePD[CH24]=<I8>\r\nchannelPercentagePD[CH25]=<I8>\r\nchannelPercentagePD[CH26]=<I8>" "<NONE>" "RampTime=<U16>" "<NONE>" "<NONE>" "address=<U32>\r\nlength=<U16>" "address=<U32>\r\nlength=<U16>" "<NONE>" "<NONE>" "<NONE>" "<NONE>" "command(0=Read,1=Clear)\nselect(0=Capacitor,1=Impedance,2=Vbat,3=Thermistor)" "bgiAmplitude=0\r\nenabled(0=Enabled,1=Disabled)" "<NONE>"] -> w3
    frame 0, Default {
    }
    frame 1 {
      # "Get xPG Status"
    }
    frame 2 {
      # "Stimulation"
    }
    frame 3 {
      # "Select Program"
    }
    frame 4 {
      # "Increment Program Amplitude"
    }
    frame 5 {
      # "Decrement Program Amplitude"
    }
    frame 6 {
      # "Get PoP Constants"
    }
    frame 7 {
      # "Get PPC Constants"
    }
    frame 8 {
      # "Get Program Names"
    }
    frame 9 {
      # "Set Pulse Amplitude"
    }
    frame 10 {
      # "Increment Pulse Amplitude"
    }
    frame 11 {
      # "Decrement Pulse Amplitude"
    }
    frame 12 {
      # "Get Pulse Widths"
    }
    frame 13 {
      # "Set Pulse Widths"
    }
    frame 14 {
      # "Increment Pulse Width"
    }
    frame 15 {
      # "Decrement Pulse Width"
    }
    frame 16 {
      # "Get Program Frequency"
    }
    frame 17 {
      # "Set Program Frequency"
    }
    frame 18 {
      # "Increment Program Frequency"
    }
    frame 19 {
      # "Decrement Program Frequency"
    }
    frame 20 {
      # "Inject Event"
    }
    frame 21 {
      # "Charging Control"
    }
    frame 22 {
      # "Get xPG Identity"
    }
    frame 23 {
      # "Set xPG Identity"
    }
    frame 24 {
      # "Restore Program Defaults"
    }
    frame 25 {
      # "Get Program Definition"
    }
    frame 26 {
      # "Set Program Definition"
    }
    frame 27 {
      # "Get Program Constants"
    }
    frame 28 {
      # "Set Program Constants"
    }
    frame 29 {
      # "Get Configurable Device Parameters"
    }
    frame 30 {
      # "Set Configurable Device Parameters"
    }
    frame 31 {
      # "Get Pulse Constants"
    }
    frame 32 {
      # "Set Pulse Constants"
    }
    frame 33 {
      # "Get Lead Limits"
    }
    frame 34 {
      # "Set Lead Limits"
    }
    frame 35 {
      # "Get Channel Calibrations"
    }
    frame 36 {
      # "Set Channel Calibrations"
    }
    frame 43 {
      # "Get Stim ASIC HV Calibrations"
    }
    frame 44 {
      # "Set Stim ASIC HV Calibrations"
    }
    frame 47 {
      # "Get CP Data Block"
    }
    frame 48 {
      # "Set CP Data Block"
    }
    frame 49 {
      # "Clear Log"
    }
    frame 50 {
      # "Read Log"
    }
    frame 51 {
      # "Append Log"
    }
    frame 52 {
      # "Get Patient Program Run-Time"
    }
    frame 53 {
      # "Set Program Run-Time"
    }
    frame 54 {
      # "Impedance Measurement"
    }
    frame 55 {
      # "Enter Storage Mode"
    }
    frame 56 {
      # "Echo Short (use CP Data)"
    }
    frame 57 {
      # "Echo Long (use CP Data)"
    }
    frame 58 {
      # "Get General Calibration"
    }
    frame 59 {
      # "Set General Calibration"
    }
    frame 60 {
      # "Get Trim List"
    }
    frame 61 {
      # "Set Trim List"
    }
    frame 62 {
      # "Get Counter"
    }
    frame 63 {
      # "Set Counter"
    }
    frame 64 {
      # "Get Test Stimulation"
    }
    frame 65 {
      # "Set Test Stimulation"
    }
    frame 66 {
      # "Get Titration Stimulation"
    }
    frame 67 {
      # "Set Titration Stimulation"
    }
    frame 68 {
      # "Get Ramp Time"
    }
    frame 69 {
      # "Set Ramp Time"
    }
    frame 70 {
      # "Get VBAT"
    }
    frame 71 {
      # "Set Software Description Block"
    }
    frame 72 {
      # "Pending"
      # "Write Memory"
    }
    frame 73 {
      # "Read Memory"
    }
    frame 74 {
      # "Reset xPG"
    }
    frame 75 {
      # "Erase Flash Block"
    }
    frame 76 {
      # "Write Vectors"
    }
    frame 77 {
      # "Read Vectors"
    }
    frame 78 {
      # "Diagnostic Data"
    }
    frame 79 {
      # "Set Background Impedance"
    }
    frame 80 {
      # "Get Background Impedence"
    }
  }
  "Template String" <- w3
